vi "Thingworx_Write.vi"(8 "error in (no error)":errorcluster, 10 "Property In":T3, 11 "Device in":T2) -> (0 "error out":errorcluster, 1 "Comm":T1, 3 "Device Out out":T2)   [LabVIEW 2016]
uses:
  _subVIs/Device.ctl
  _subVIs/HTTPComm.ctl
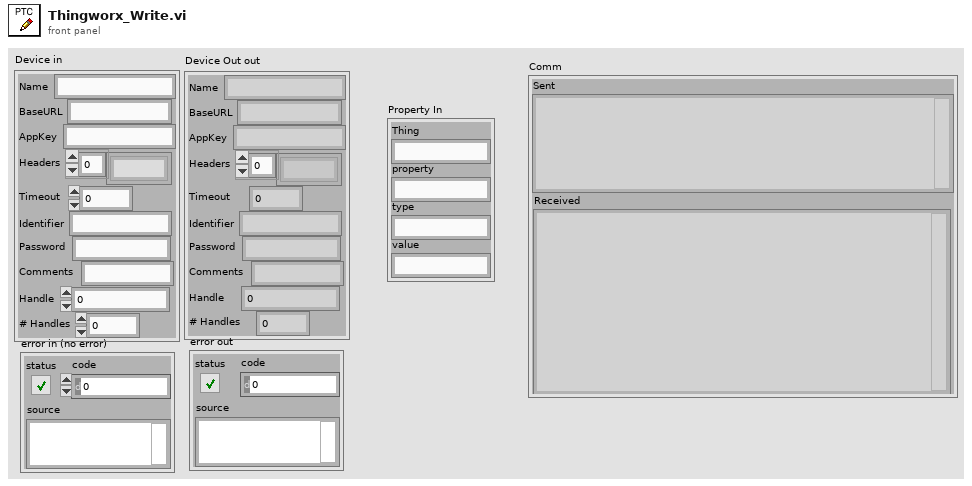
[diagram p1: front panel]
types:
  T1 = typedef "HTTPComm.ctl" = cluster{"url":string, "sent headers":string, "sent body":string, "headers":string, "body":string, "Sent":string, "Received":string}
  T2 = typedef "Device.ctl" = cluster{"Name":string, "BaseURL":string, "AppKey":string, "Headers":string[], "Timeout":i32, "Identifier":string, "Password":string, "Comments":string, "Handle":u32, "# Handles":i32}
  T3 = cluster{"Thing":string, "property":string, "type":string, "value":string}
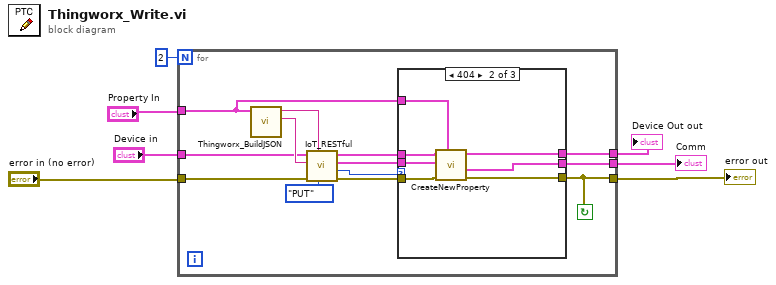
[diagram p0: block diagram]
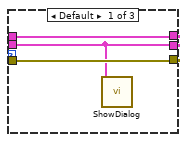
[diagram p2: hidden frame]
diagram:
  n1 = for {
    N: 2 -> [_]
    tunnel: "Property In" -> [w14]
    tunnel: "error in (no error)" -> [w15]
    tunnel: [w9] -> w2
    tunnel: "Device in" -> [w12]
    tunnel: [w11] -> w3
    tunnel: [w8] -> w1
    stop <- w9 continue-if-true
    n2 = call "Thingworx_BuildJSON.vi"("Property In"=w14) -> ("JSON"=w20:string, "URL"=w18:string)  [unwired: 9 in]
    n3 = call "IoT_RESTful.vi"("Method"=enum16{"GET", "PUT", "POST", "MultiPOST"}."PUT", "url"=w18, "error in"=w15, "JSON"=w20, "Device In"=w12) -> ("error out"=w10:errorcluster, "HTTP Code"=w17:i32, "Comm"=w16:T1, "Device Out"=w13:T2)  [unwired: 3 in]
    n4 = case shown="404" w17 {
      tunnel: w16 -> [w21 w26 w31]
      tunnel: w14 -> [_ w24 _]
      tunnel: w13 -> [w23 w30 w33]
      tunnel: [w23 w29 w33] -> w11
      tunnel: w10 -> [w22 w28 w32]
      tunnel: [w22 w27 w32] -> w9
      tunnel: [w21 w25 w31] -> w8
      frame Default {
        n5 = call "ShowDialog.vi"("Comm"=w21) -> ()  [unwired: 11 in]
      }
      frame 404 {
        n6 = call "CreateNewProperty.vi"("Property In"=w24, "error in"=w28, "Comm  In"=w26, "Device In"=w30) -> ("error out"=w27:errorcluster, "Comm Out"=w25:T1, "Device Out"=w29:T2)  [unwired: 5 in]
      }
      frame 200 {
      }
    }
  }
  "Device Out out" <- w3
  "error out" <- w2
  "Comm" <- w1
